vi "TransformationMatrix.vi"   [LabVIEW 2014]
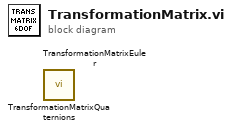
[diagram p0: block diagram]
diagram:
  n1 = call "TransformationMatrixQuaternions.vi"() -> ()  [unwired: 1 in, 1 out]
  n2 = call "TransformationMatrixEuler.vi"() -> ()  [unwired: 1 in, 1 out]
